vi "Add_Update_Values.vi"(0 "Filename":path, 1 "Value  Constant?":bool, 2 "Edit Raw data files?":bool, 3 "Filetype":string, 5 "New Chs In":string[](array[string])=[""], 7 "Edit Raw Data Header Info":bool, 9 "New Values In":string[][](array[string]), 11 "Selected Rows":i32[](array[numeric]), 12 "Edit all Rows?":bool, 13 "Raw DF in Orig Pos?":bool, 14 "Job Directory":path=path "/G4_2_HD/Users/paulhayden/Documents/Projects/Hong Roughness/XW data/XW_Corr.tpt") -> ()   [LabVIEW 2010]
panel:
  in  "Warn If files not found?":bool=TRUE
  out "Checking Raw data files":i32
  in  "stop":bool
  out "Currently editing":string
  out "Folder Containing Raw data Files":path
  out "size(s)":i32
  out "Files Processed":i32(slide) scale=0.0..6249.0
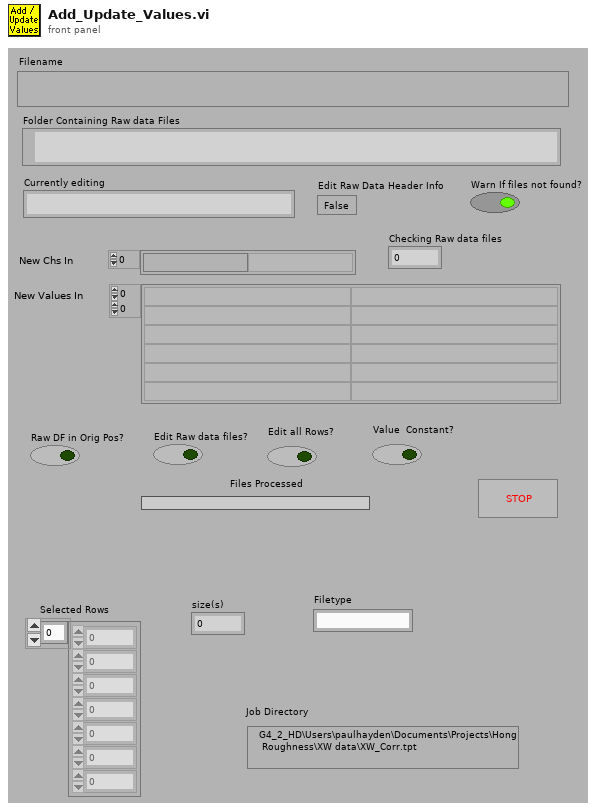
[diagram p1: front panel]
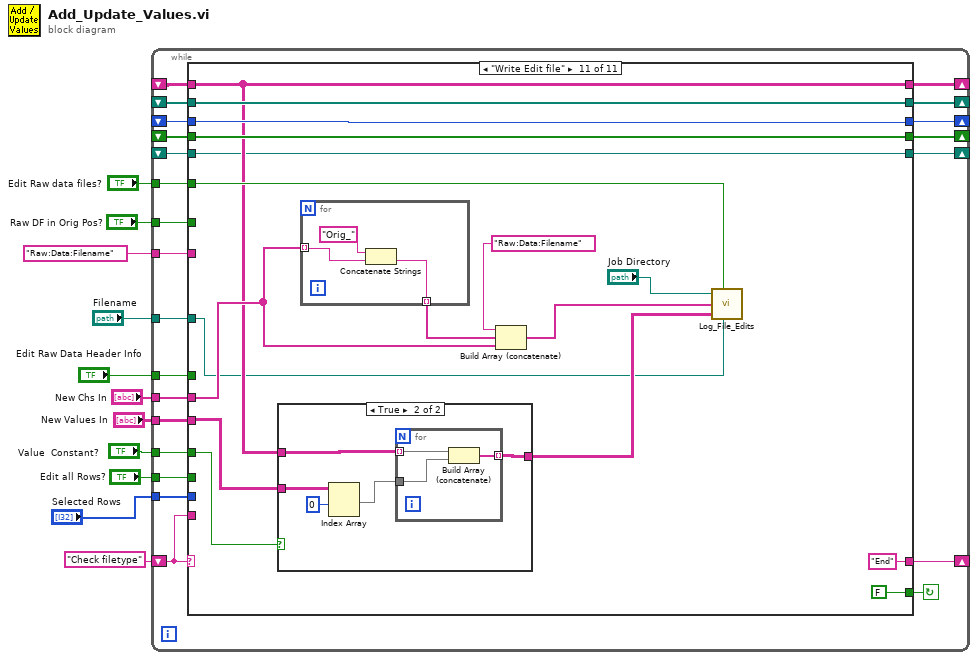
[diagram p0: block diagram]
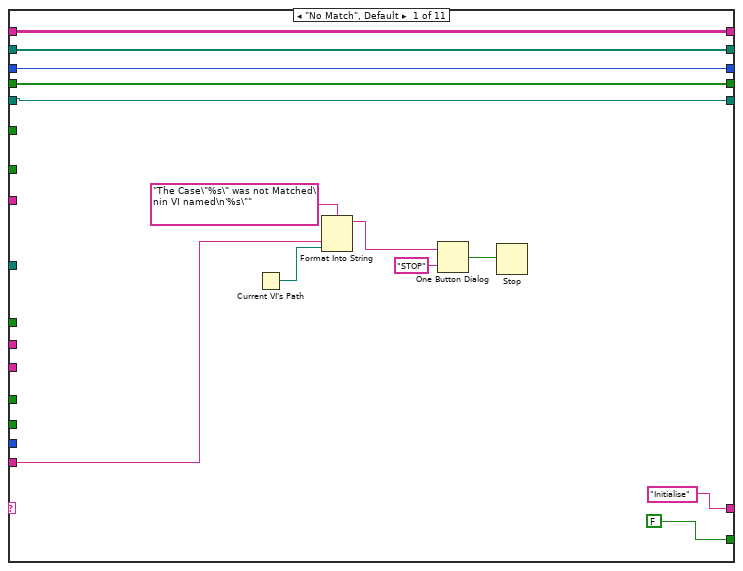
[diagram p2: hidden frame]
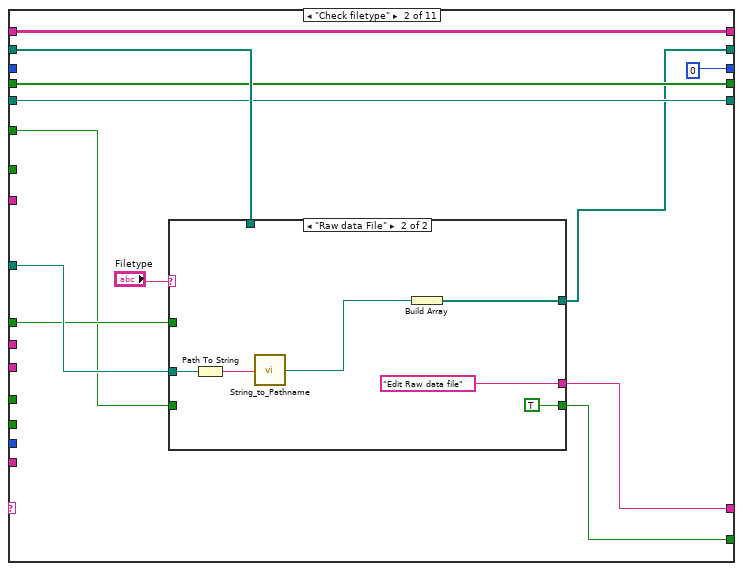
[diagram p3: hidden frame]
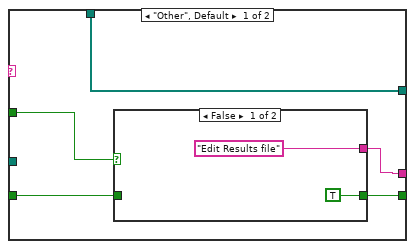
[diagram p4: hidden frame]
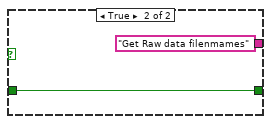
[diagram p5: hidden frame]
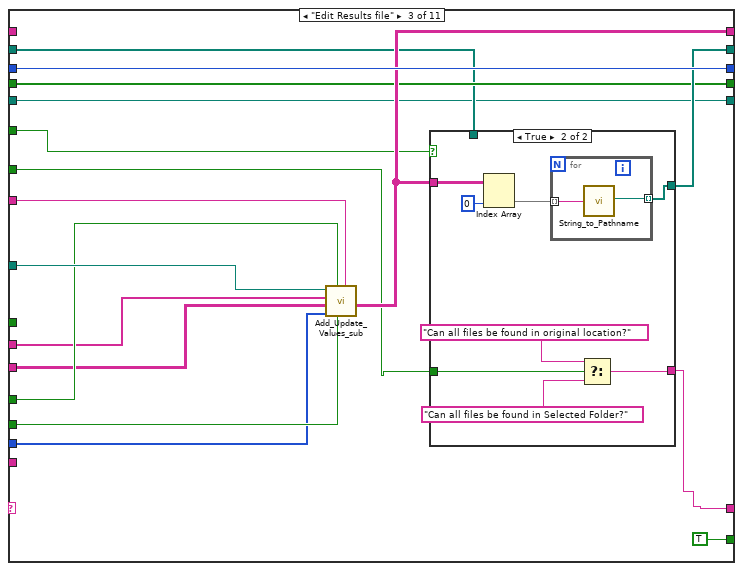
[diagram p6: hidden frame]
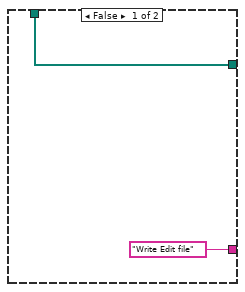
[diagram p7: hidden frame]
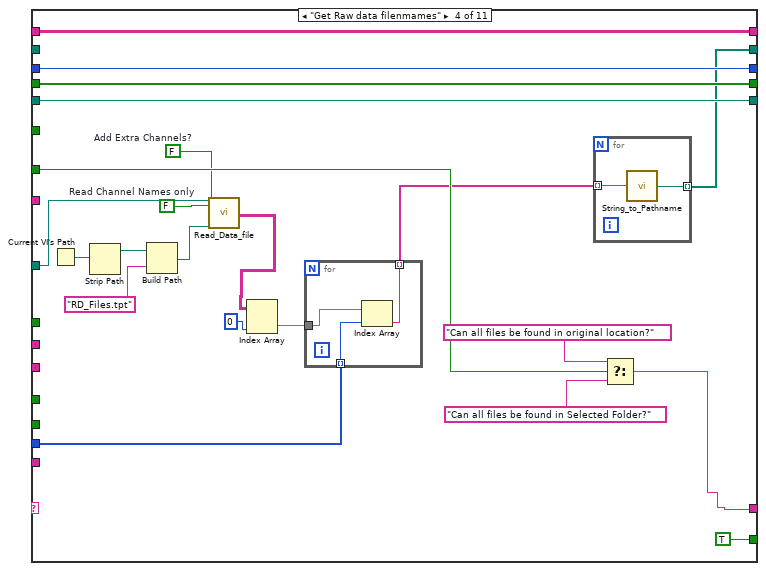
[diagram p8: hidden frame]
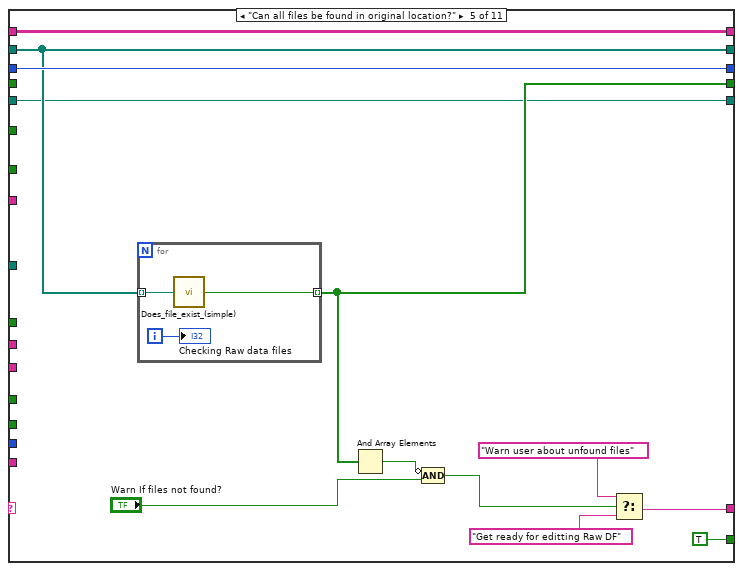
[diagram p9: hidden frame]
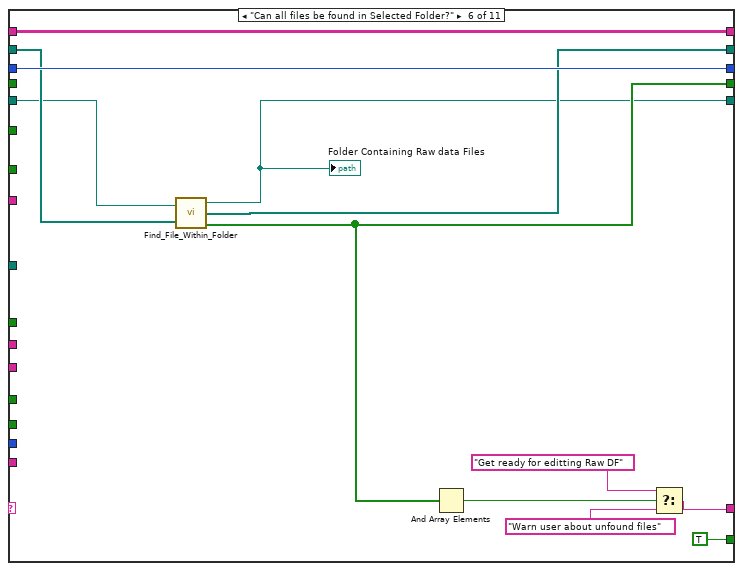
[diagram p10: hidden frame]
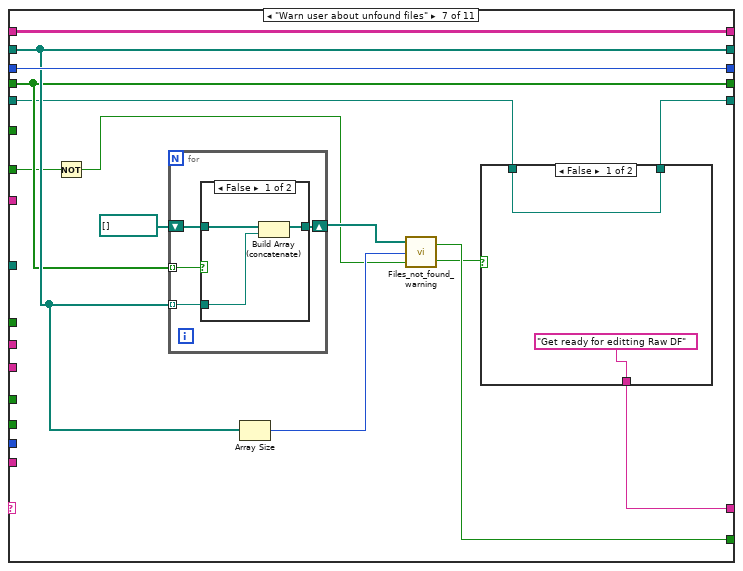
[diagram p11: hidden frame]
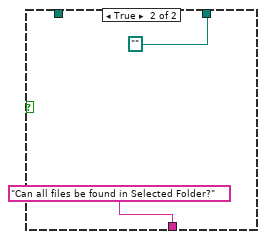
[diagram p12: hidden frame]
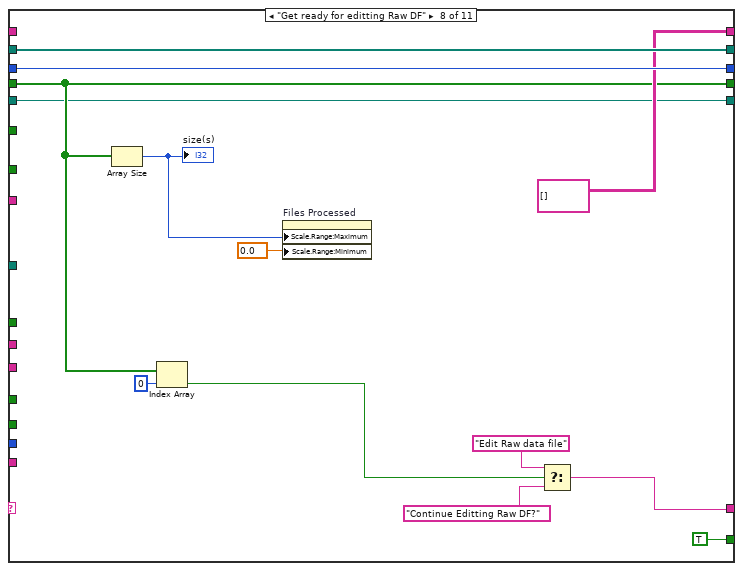
[diagram p14: hidden frame]
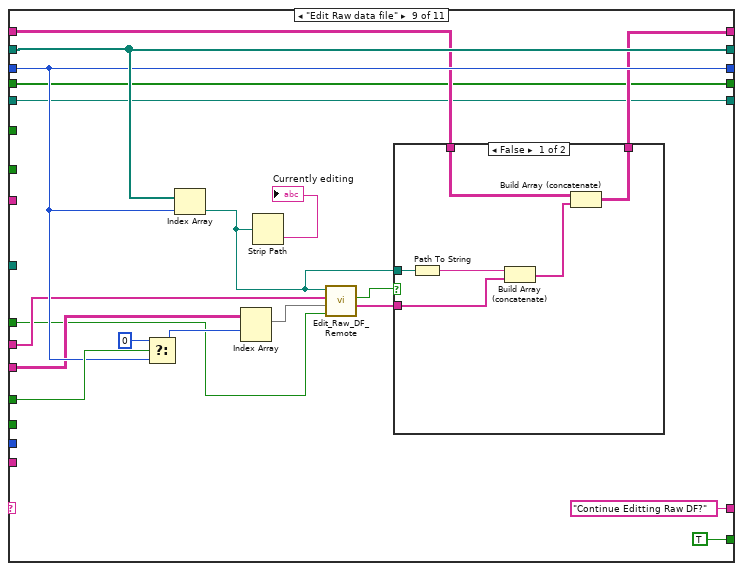
[diagram p15: hidden frame]
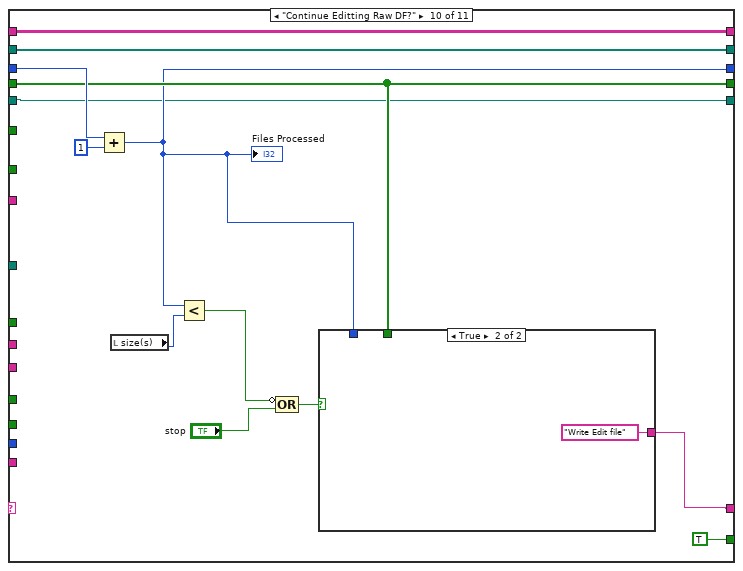
[diagram p17: hidden frame]
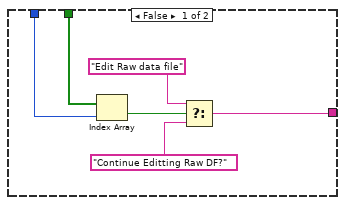
[diagram p18: hidden frame]
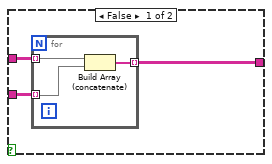
[diagram p19: hidden frame]
diagram:
  n1 = while {
    shift-left: "Check filetype" -> [w32]
    shift-right: [w33] -> _
    shift-right: [w30] -> _
    shift-left: _ -> [w29]
    tunnel: "Filename" -> [w31]
    shift-right: [w28] -> _
    shift-left: _ -> [w27]
    tunnel: "Value  Constant?" -> [w26]
    tunnel: "Edit Raw Data Header Info" -> [w25]
    shift-right: [w24] -> _
    shift-left: _ -> [w23]
    tunnel: "New Chs In" -> [w22]
    tunnel: "New Values In" -> [w21]
    tunnel: "Edit all Rows?" -> [w20]
    shift-right: [w19] -> _
    shift-left: _ -> [w18]
    tunnel: "Edit Raw data files?" -> [w17]
    tunnel: "Raw DF in Orig Pos?" -> [w16]
    shift-right: [w14] -> _
    shift-left: _ -> [w15]
    tunnel: "Selected Rows" -> [w13]
    tunnel: "Raw:Data:Filename" -> [w12]
    stop <- w34 continue-if-true
    n2 = case shown="\"Write Edit file\"" w32 {
      tunnel: [FALSE w50 TRUE TRUE TRUE TRUE w165 TRUE TRUE TRUE FALSE] -> w34
      tunnel: ["Initialise" w57 w80 w122 w137 w148 w161 w188 "Continue Editting Raw DF?" ("t") w227 "End" ("t")] -> w33
      tunnel: w32 -> [w42 _ _ _ _ _ _ _ _ _ _]
      tunnel: w31 -> [_ w55 w89 w111 _ _ _ _ _ _ w245]
      tunnel: [w38 w48 w83 w105 w140 w154 w167 w194 w212 w233 w258] -> w30
      tunnel: w29 -> [w38 w58 w79 _ w140 w153 w167 w194 w212 w233 w258]
      tunnel: [w39 0 w91 w125 w142 w157 w171 w196 w211 w228 w256] -> w28
      tunnel: w27 -> [w39 _ w91 w125 w142 w157 w171 w196 w211 w232 w256]
      tunnel: w26 -> [_ _ w88 _ _ _ _ _ w215 _ w246]
      tunnel: w25 -> [_ w51 _ _ _ _ _ _ w197 _ _]
      tunnel: [w37 w54 w84 w117 w139 w155 w169 string[][] [] ("Edit Info") w202 w234 w249] -> w24
      tunnel: w23 -> [w37 w54 _ w117 w139 w155 w169 _ w203 w234 w249]
      tunnel: w22 -> [_ _ w87 _ _ _ _ _ w209 _ w251]
      tunnel: w21 -> [_ _ w86 _ _ _ _ _ w208 _ w248]
      tunnel: w20 -> [_ _ w85 _ _ _ _ _ _ _ _]
      tunnel: [w36 w53 w82 w123 w138 w149 w166 w192 w201 w229 w257] -> w19
      tunnel: w18 -> [w36 w53 w82 w123 _ _ w166 w192 w201 w229 w257]
      tunnel: w17 -> [_ w49 w81 _ _ _ _ _ _ _ w253]
      tunnel: w16 -> [_ _ w78 w121 _ _ w164 _ _ _ _]
      tunnel: w15 -> [w35 w52 w77 w120 w136 w147 w158 w184 w198 w223 w243]
      tunnel: [w35 w52 w77 w120 w136 w146 w159 w184 w198 w223 w243] -> w14
      tunnel: w13 -> [_ _ w76 w116 _ _ _ _ _ _ _]
      tunnel: w12 -> [_ _ w75 _ _ _ _ _ _ _ _]
      frame "No Match", Default {
        n3 = Current VI's Path() -> (path=w41:path)
        n4 = Format Into String(format string="The Case\"%s\" was not Matched\nin VI named\n'%s\"" ("Format String"), w42, w41) -> (resulting string=w45:string)  [unwired: 2 in, 1 out]
        n5 = One Button Dialog(message=w45, button name ("OK")="STOP") -> (true=w43:bool)
        n6 = Stop(stop? (T)=w43) -> ()
      }
      frame "Check filetype" {
        n7 = case shown="\"Raw data File\"" "Filetype" {
          tunnel: w55 -> [_ w71]
          tunnel: [w64 w74] -> w48
          tunnel: w58 -> [w64 _]
          tunnel: [w62 "Edit Raw data file"] -> w57
          tunnel: w51 -> [w63 _]
          tunnel: [w61 TRUE ("Edit Raw data files?")] -> w50
          tunnel: w49 -> [w60 _]
          frame "Other", Default {
            n8 = case shown="False" w63 {
              tunnel: ["Edit Results file" "Get Raw data filenmames"] -> w62
              tunnel: [TRUE ("Edit Raw data files?") w67] -> w61
              tunnel: w60 -> [_ w67]
              frame False {
              }
              frame True {
              }
            }
          }
          frame "Raw data File" {
            n9 = Path To String(path=w71) -> (string=w70:string)
            n10 = call "String_to_Pathname.vi"("Input String"=w70) -> ("path"=w69:path)
            n11 = Build Array(w69) -> (w74:path[])
          }
        }
      }
      frame "Edit Results file" {
        n12 = call "Add_Update_Values_sub.vi"("Raw data Filename column name"=w75, "Edit all Rows?"=w85, "Value  Constant?"=w88, "Selected Rows"=w76, "New Values In"=w86, "New Chs In"=w87, "Filename"=w89) -> ("Edit Info"=w84:string[][])  [unwired: 4 out]
        n13 = case shown="True" w81 {
          tunnel: w84 -> [_ w101]
          tunnel: [w92 w95] -> w83
          tunnel: w78 -> [_ w99]
          tunnel: ["Write Edit file" w96] -> w80
          tunnel: w79 -> [w92 _]
          frame False {
          }
          frame True {
            n14 = Index Array(array=w101, index (col)=0 ("disabled index (col)")) -> (element=w94:string[])  [unwired: 1 in]
            n15 = for {
              tunnel: [w102] -> w95 mode=indexing
              tunnel: w94 -> [w103] mode=indexing
              n16 = call "String_to_Pathname.vi"("Input String"=w103) -> ("path"=w102:path)
            }
            n17 = Select(t="Can all files be found in original location?", s=w99, f="Can all files be found in Selected Folder?") -> (s? t:f=w96:string)
          }
        }
      }
      frame "Get Raw data filenmames" {
        w108 = FALSE  # Add Extra Channels?
        w109 = FALSE  # Read Channel Names only
        n18 = Current VI's Path() -> (path=w114:path)
        n19 = Strip Path(path=w114) -> (stripped path=w113:path)  [unwired: 1 out]
        n20 = Build Path(base path=w113, name or relative path="RD_Files.tpt") -> (appended path=w110:path)
        n21 = call "Read_Data_file.vi"("Results file"=w111, "Read Channel Names only"=w109, "Add Extra Channels?"=w108, "Template File"=w110) -> ("Channel Values Out"=w107:string[][])  [unwired: 1 in, 14 out]
        n22 = Index Array(array=w107, index (col)=0 ("index (row)")) -> (element=w115:string[])  [unwired: 1 in]
        n23 = for {
          tunnel: w116 -> [w130] mode=indexing
          tunnel: w115 -> [w129]
          tunnel: [w128] -> w104 mode=indexing
          n24 = Index Array(array=w129, index=w130) -> (element=w128:string)
        }
        n25 = for {
          tunnel: [w127] -> w105 mode=indexing
          tunnel: w104 -> [w126] mode=indexing
          n26 = call "String_to_Pathname.vi"("Input String"=w126) -> ("path"=w127:path)
        }
        n27 = Select(t="Can all files be found in original location?", s=w121, f="Can all files be found in Selected Folder?") -> (s? t:f=w122:string)
      }
      frame "Can all files be found in original location?" {
        n28 = for {
          tunnel: w140 -> [w145] mode=indexing
          tunnel: [w144] -> w138 mode=indexing
          i -> [w143]
          n29 = call "Does_file_exist_(simple).vi"("Pathname"=w145) -> ("exists?"=w144:bool)
          "Checking Raw data files" <- w143
        }
        n30 = And Array Elements(Boolean array=w138) -> (logical AND=w135:bool)
        n31 = Compound Arithmetic op=AND(invert w135, "Warn If files not found?") -> (w133:bool)
        n32 = Select(t="Warn user about unfound files", s=w133, f="Get ready for editting Raw DF" ("t")) -> (s? t:f=w137:string)
      }
      frame "Can all files be found in Selected Folder?" {
        n33 = call "Find_File_Within_Folder.vi"("Folder to Search"=w147, "Files to find"=w153) -> ("Folder to Search Out"=w146:path, "New File Paths"=w154:path[], "Files Found?"=w149:bool[])
        "Folder Containing Raw data Files" <- w146
        n34 = And Array Elements(Boolean array=w149) -> (logical AND=w152:bool)
        n35 = Select(t="Get ready for editting Raw DF", s=w152, f="Warn user about unfound files") -> (s? t:f=w148:string)
      }
      frame "Warn user about unfound files" {
        n36 = Not(x=w164) -> (.not. x?=w163:bool)
        n37 = for {
          tunnel: w167 -> [w176] mode=indexing
          shift-right: [w179] -> w168
          shift-left: path[] [] -> [w178]
          tunnel: w166 -> [w177] mode=indexing
          n38 = case shown="False" w177 {
            tunnel: w178 -> [w182 w183]
            tunnel: [w180 w183] -> w179
            tunnel: w176 -> [w181 _]
            frame False {
              n39 = Build Array (concatenate)(w182, w181) -> (w180:path[])
            }
            frame True {
            }
          }
        }
        n40 = Array Size(array=w167) -> (size(s)=w170:i32)
        n41 = call "Files_not_found_warning.vi"("Use Selected Folder?"=w163, "Total number of data files"=w170, "Unfound Files"=w168) -> ("Edit Selected Folder Out"=w162:bool, "Edit Files?"=w165:bool)
        n42 = case shown="False" w162 {
          tunnel: ["Get ready for editting Raw DF" ("t") "Can all files be found in Selected Folder?" ("t")] -> w161
          tunnel: [w172 path ""] -> w159
          tunnel: w158 -> [w172 _]
          frame False {
          }
          frame True {
          }
        }
      }
      frame "Get ready for editting Raw DF" {
        n43 = Array Size(array=w192) -> (size(s)=w185:i32)
        "size(s)" <- w185
        n44 = Index Array(array=w192, index=0) -> (element=w190:bool)
        n45 = property on="Files Processed" class="Slide (strict)"("Scale.Range:Maximum"=w185, "Scale.Range:Minimum"=0.0 ("Scale.Range:Maximum")) -> ()  [unwired: 2 in, 2 out]
        n46 = Select(t="Edit Raw data file", s=w190, f="Continue Editting Raw DF?") -> (s? t:f=w188:string)
      }
      frame "Edit Raw data file" {
        n47 = Select(t=0, s=w215, f=w211) -> (s? t:f=w213:i32)
        n48 = Index Array(array=w212, index=w211) -> (element=w200:path)
        n49 = Index Array(array=w208, index (row)=w213) -> (element=w207:string[])  [unwired: 1 in]
        n50 = Strip Path(path=w200) -> (name=→"Currently editing":string)  [unwired: 1 out]
        n51 = call "Edit_Raw_DF_Remote.vi"("Edit Raw Data Header Info"=w197, "New Values In"=w207, "New Chs In"=w209, "Current Filename"=w200) -> ("Original values"=w205:string[], "File Not Changed?"=w204:bool)  [unwired: 2 out]
        n52 = case shown="False" w204 {
          tunnel: w200 -> [w221 _]
          tunnel: w205 -> [w219 _]
          tunnel: w203 -> [w217 w222]
          tunnel: [w216 w222] -> w202
          frame False {
            n53 = Path To String(path=w221) -> (string=w220:string)
            n54 = Build Array (concatenate)(w220, w219) -> (w218:string[])
            n55 = Build Array (concatenate)(w217, w218) -> (w216:string[][])
          }
          frame True {
          }
        }
      }
      frame "Continue Editting Raw DF?" {
        n56 = Add(x=w232, y=1) -> (x+y=w228:i32)
        "Files Processed" <- w228
        n57 = local read "size(s)"() -> (w230:i32)
        n58 = Less?(x=w228, y=w230) -> (x < y?=w225:bool)
        n59 = Compound Arithmetic op=OR(invert w225, "stop") -> (w224:bool)
        n60 = case shown="True" w224 {
          tunnel: w229 -> [w240 _]
          tunnel: w228 -> [w239 _]
          tunnel: [w237 "Write Edit file" ("t")] -> w227
          frame False {
            n61 = Index Array(array=w240, index=w239) -> (element=w241:bool)
            n62 = Select(t="Edit Raw data file", s=w241, f="Continue Editting Raw DF?") -> (s? t:f=w237:string)
          }
          frame True {
          }
        }
      }
      frame "Write Edit file" {
        n63 = case shown="True" w246 {
          tunnel: w249 -> [w262 w270]
          tunnel: w248 -> [w261 w268]
          tunnel: [w260 w269] -> w247
          frame False {
            n64 = for {
              tunnel: w262 -> [w265] mode=indexing
              tunnel: w261 -> [w264] mode=indexing
              tunnel: [w263] -> w260 mode=indexing
              n65 = Build Array (concatenate)(w265, w264) -> (w263:string[])
            }
          }
          frame True {
            n66 = Index Array(array=w268, index (row)=0) -> (element=w266:string[])  [unwired: 1 in]
            n67 = for {
              tunnel: w270 -> [w273] mode=indexing
              tunnel: [w272] -> w269 mode=indexing
              tunnel: w266 -> [w271]
              n68 = Build Array (concatenate)(w273, w271) -> (w272:string[])
            }
          }
        }
        n69 = for {
          tunnel: w251 -> [w276] mode=indexing
          tunnel: [w274] -> w252 mode=indexing
          n70 = Concatenate Strings("Orig_" ("string"), w276) -> (w274:string)
        }
        n71 = Build Array (concatenate)("Raw:Data:Filename", w252, w251) -> (w250:string[])
        n72 = call "Log_File_Edits.vi"("Job Directory"="Job Directory", "File Editted?"=w253, "Channels to Edit"=w250, "Data"=w247, "Results file name"=w245) -> ()  [unwired: 2 out]
      }
    }
  }
